vi "set_subpanel_reference.vi"(8 "error in (no error)":errorcluster, 10 "Sub Panel":refnum<vi>, 11 "simple_html_chat_ui in":refnum<class "simple_html_chat_ui.lvclass">) -> (0 "error out":errorcluster, 3 "simple_html_chat_ui out":refnum<class "simple_html_chat_ui.lvclass">)   [LabVIEW 2020, in "simple_html_chat_ui.lvclass"]
uses:
  simple_html_chat_ui.lvclass
  typedefs/ui_user_event.ctl
  simple_html_chat_ui.lvclass/simple_html_chat_ui.ctl
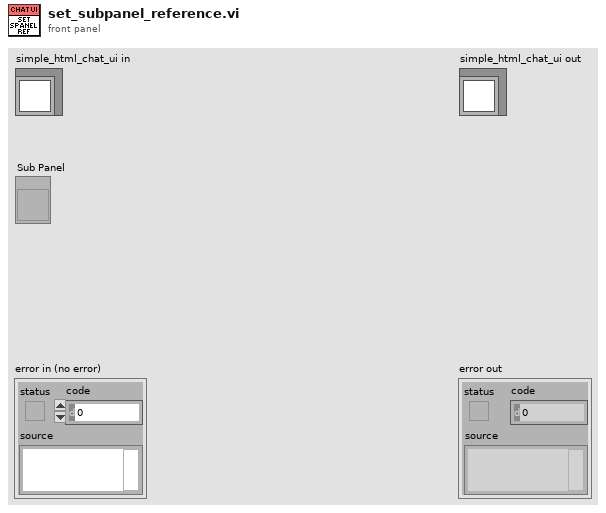
[diagram p1: front panel]
types:
  T1 = typedef "simple_html_chat_ui.lvclass/ui_user_event.ctl" = enum16{"Initialize", "Generate", "Get Reference", "Destroy"}
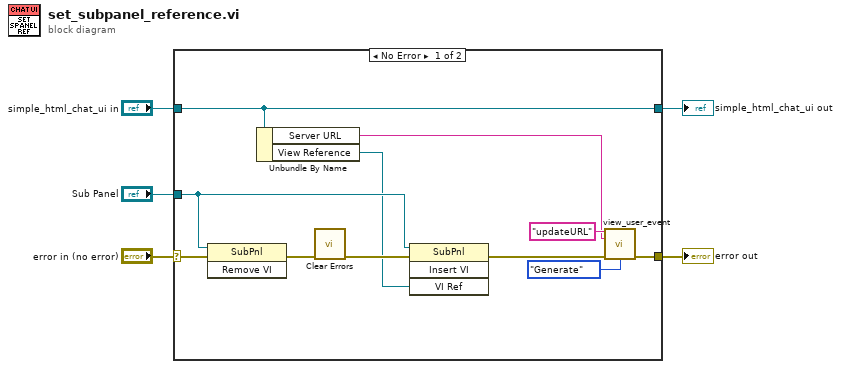
[diagram p0: block diagram]
diagram:
  n1 = case shown="No Error" "error in (no error)" {
    selector: "error in (no error)" -> [w14 w18]
    tunnel: [w7 w18] -> w4
    tunnel: [w12 w17] -> w2
    tunnel: "simple_html_chat_ui in" -> [w12 w17]
    tunnel: "Sub Panel" -> [w13 _]
    frame No Error {
      n2 = invoke class="SubPnl" method="Remove VI"(reference=w13, error in=w14) -> (error out=w16:errorcluster)  [unwired: 1 in, 2 out]
      n3 = Unbundle By Name(w12) -> ("Server URL"=w6:string, "View Reference"=w11:refnum<vi>)
      n4 = call <vilib>:"Clear Errors.vi"("error in (no error)"=w16) -> ("error out"=w15:errorcluster)  [unwired: 5 in, 1 out]
      n5 = invoke class="SubPnl" method="Insert VI"(reference=w13, error in=w15, "VI Ref"=w11) -> (error out=w8:errorcluster)  [unwired: 1 in, 3 out]
      n6 = call "view_user_event.vi"("State"="updateURL", "Data"=w6, "error in (no error)"=w8, "Operation"=ui_user_event."Generate") -> ("error out"=w7:errorcluster)  [unwired: 10 in, 1 out]
    }
    frame Error {
    }
  }
  "error out" <- w4
  "simple_html_chat_ui out" <- w2
